vi "To Serial Form.vi"(6 "Serial Version":T1, 10 "Serializer in":refnum<class "Serializer.lvclass">, 11 "PAS Data in":refnum<class "PAS Data.lvclass">) -> (0 "error out":errorcluster, 2 "Serializer out":refnum<class "Serializer.lvclass">, 3 "PAS Data out":refnum<class "PAS Data.lvclass">)   [LabVIEW 2014, in "PAS Data.lvclass"]
uses:
  PAS Data.lvclass
  <vilib>/NI/AQ Character Lineator/Serializer/Serializer.lvclass
  <vilib>/NI/AQ Character Lineator/Serialization Common/Serial Version.ctl
  Cell/PAS Cell Data.lvclass
  PAS Data.lvclass/PAS Data.ctl
  <vilib>/NI/AQ Character Lineator/Serializable/Insert Serializable Array.vi
  <vilib>/NI/AQ Character Lineator/Serializable/Insert Timestamp.vi
  <vilib>/NI/AQ Character Lineator/Serializable/Insert Boolean.vi
  <vilib>/NI/AQ Character Lineator/Serializer/Insert Timestamp.vi
  <vilib>/NI/AQ Character Lineator/Serializer/Insert Boolean.vi
  <vilib>/NI/AQ Character Lineator/Serializer/Read Include Default Values.vi
  <vilib>/NI/AQ Character Lineator/Serializer/Insert Serializable Array.vi
  Data/Data.lvclass
  <vilib>/NI/AQ Character Lineator/Serializable/Serializable.lvclass
  <vilib>/NI/AQ Character Lineator/Serialization Common/Serialization Common.lvlib
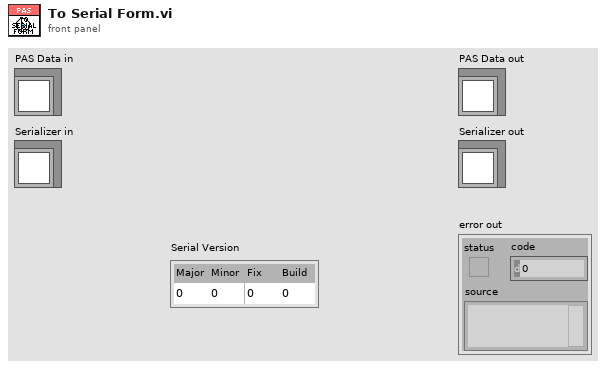
[diagram p1: front panel]
types:
  T1 = typedef "Serialization Common.lvlib/Serial Version.ctl" = cluster{"Major":u16, "Minor":u16, "Fix":u16, "Build":u16}
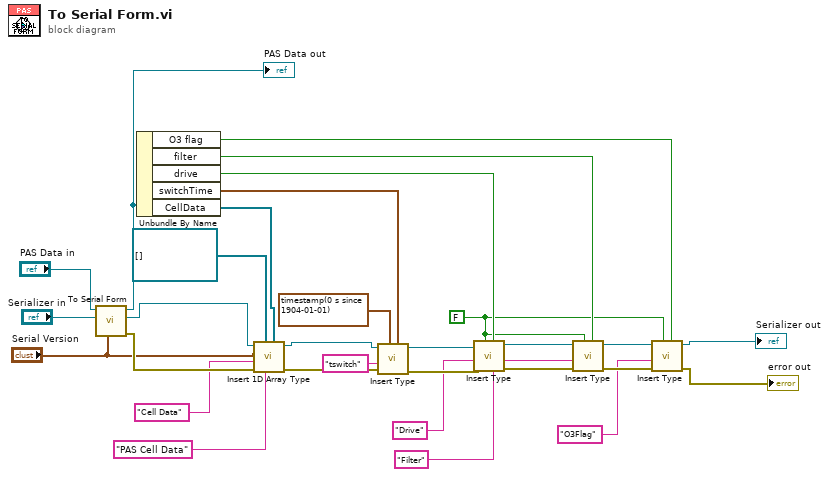
[diagram p0: block diagram]
diagram:
  w3 = FALSE ("Default Value")
  n1 = call-parent "To Serial Form.vi"("Serial Version"="Serial Version", "Serializer in"="Serializer in", "Data in"="PAS Data in") -> ("error out"=w24:errorcluster, "Serializer out"=w28:refnum<class "Serializer.lvclass">, "Data out"=w27:refnum<class "PAS Data.lvclass">)  [unwired: 6 in]
  "PAS Data out" <- w27
  n2 = Unbundle By Name(w27) -> ("O3 flag"=w4:bool, "filter"=w8:bool, "drive"=w13:bool, "switchTime"=w18:timestamp, "CellData"=w26:refnum<class "PAS Cell Data.lvclass">[])
  n3 = call-poly <vilib>:"Insert 1D Array Type.vi"("Serializables"=w26, "Default Class Qualified Name"="PAS Cell Data", "Default Value"=refnum<class "PAS Cell Data.lvclass">[] [] ("CellData"), "error in (no error)"=w24, "Name"="Cell Data", "Serial Version"="Serial Version", "Serializer in"=w28) -> ("error out"=w19:errorcluster, "Serializer out"=w20:refnum<class "Serializer.lvclass">)  [unwired: 3 in]
  n4 = call-poly <vilib>:"Insert Type.vi"("Time Stamp"=w18, "Default Value"=timestamp(0 s since 1904-01-01), "error in (no error)"=w19, "Name"="tswitch", "Serializer in"=w20) -> ("error out"=w14:errorcluster, "Serializer out"=w15:refnum<class "Serializer.lvclass">)  [unwired: 5 in]
  n5 = call-poly <vilib>:"Insert Type.vi"("Boolean"=w13, "Default Value"=w3, "error in (no error)"=w14, "Name"="Drive", "Serializer in"=w15) -> ("error out"=w10:errorcluster, "Serializer out"=w11:refnum<class "Serializer.lvclass">)  [unwired: 5 in]
  n6 = call-poly <vilib>:"Insert Type.vi"("Boolean"=w8, "Default Value"=w3, "error in (no error)"=w10, "Name"="Filter", "Serializer in"=w11) -> ("error out"=w6:errorcluster, "Serializer out"=w7:refnum<class "Serializer.lvclass">)  [unwired: 5 in]
  n7 = call-poly <vilib>:"Insert Type.vi"("Boolean"=w4, "Default Value"=w3, "error in (no error)"=w6, "Name"="O3Flag", "Serializer in"=w7) -> ("error out"=→"error out":errorcluster, "Serializer out"=→"Serializer out":refnum<class "Serializer.lvclass">)  [unwired: 5 in]
